vi "Destroy Test Executive.vi"(8 "error in (no error)":errorcluster, 11 "Test Executive Ref":refnum<data-value>) -> (0 "error out":errorcluster)   [LabVIEW 2019, in "Test Executive.lvlib" / "TestExecutive Ref.lvclass"]
uses:
  <vilib>/gpm_packages/@cs/test-executive/Source/Test Executive/TestExecutive Ref/TestExecutive Ref.lvclass
  <vilib>/gpm_packages/@cs/test-executive/Source/Test Executive/ITestExecutive/ITest Executive.lvclass
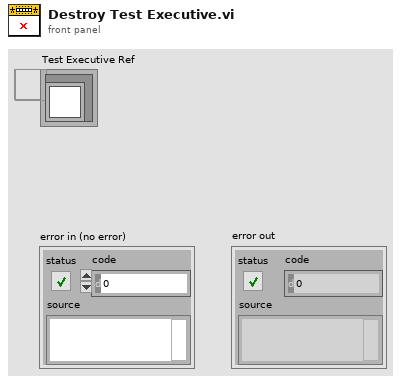
[diagram p1: front panel]
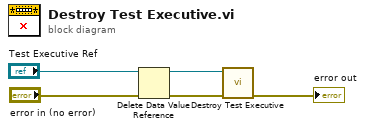
[diagram p0: block diagram]
diagram:
  n1 = Delete Data Value Reference(data value reference="Test Executive Ref", error in="error in (no error)") -> (data value=w3:refnum<class "ITest Executive.lvclass">, error out=w2:errorcluster)
  n2 = call-dynamic "Destroy Test Executive.vi"("error in (no error)"=w2, "ITest Executive in"=w3) -> ("error out"=→"error out":errorcluster)  [unwired: 9 in]
